vi "利用复数绝对值求直角三角形斜边.vi"(1 "b":dbl=4.0, 2 "a":dbl=3.0) -> (0 "c":dbl=5.0)   [LabVIEW 2012, in "几何工具.lvlib"]
doc: "功能：\n\n根据直角三角形的两个直角边a b计算斜边的长度。\n\n特点：\n\n复数的绝对值，也就是复数的幅值。\n对于a+bi,c=|a+bi|"
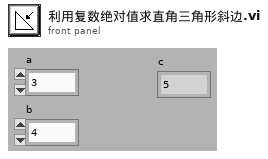
[diagram p1: front panel]
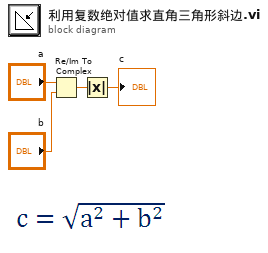
[diagram p0: block diagram]
diagram:
  n1 = Re/Im To Complex(1:"b", 2:"a") -> (0:w2:cdb)
  n2 = Absolute Value(x=w2) -> (abs(x)=→"c":dbl)
